vi "Evaluate Scope.vi"(10 "call chain":string[](array[string]), 11 "scope in":refnum<class "Scope.lvclass">) -> (2 "matches":bool[](array[boolean]), 3 "scope out":refnum<class "Scope.lvclass">)   [LabVIEW 2018, in "Logging.lvlib" / "Scope.lvclass"]
uses:
  Scope.lvclass
panel:
  # "Connector Pane"
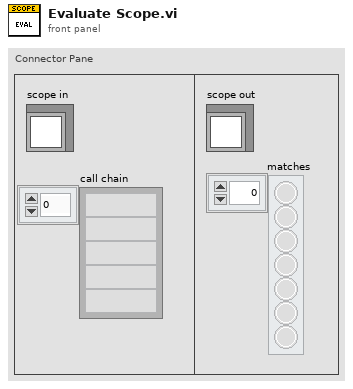
[diagram p1: front panel]
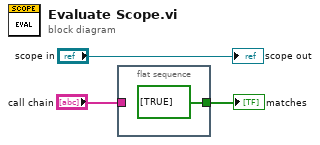
[diagram p0: block diagram]
diagram:
  n1 = flat-sequence {
    tunnel: [bool[] [TRUE] ("Boolean")] -> w3
    tunnel: "call chain" -> [_]
    frame #0 {
    }
  }
  "scope out" <- "scope in"
  "matches" <- w3
